vi "System@ErrorBox__Parameter.vi"(1 "ParamterIn":string) -> (0 "ParamterOut":string)   [LabVIEW 2020]
panel:
  in  "LogMessage":string(combo)
  in  "UserMessage":string(combo)
  in  "Logic":string(combo)
  in  "Confirm":bool
  # "System@ErrorBox $Logic,$UserMessage(,$LogMessage)"
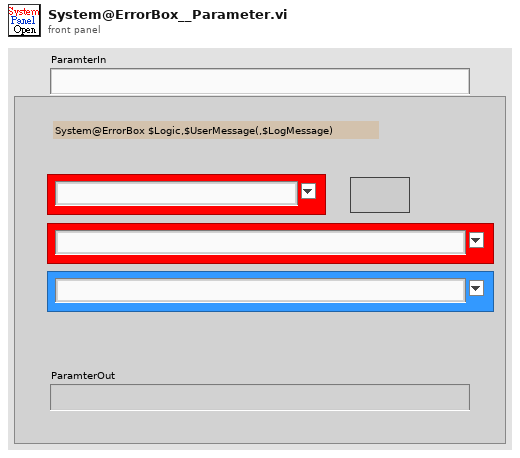
[diagram p1: front panel]
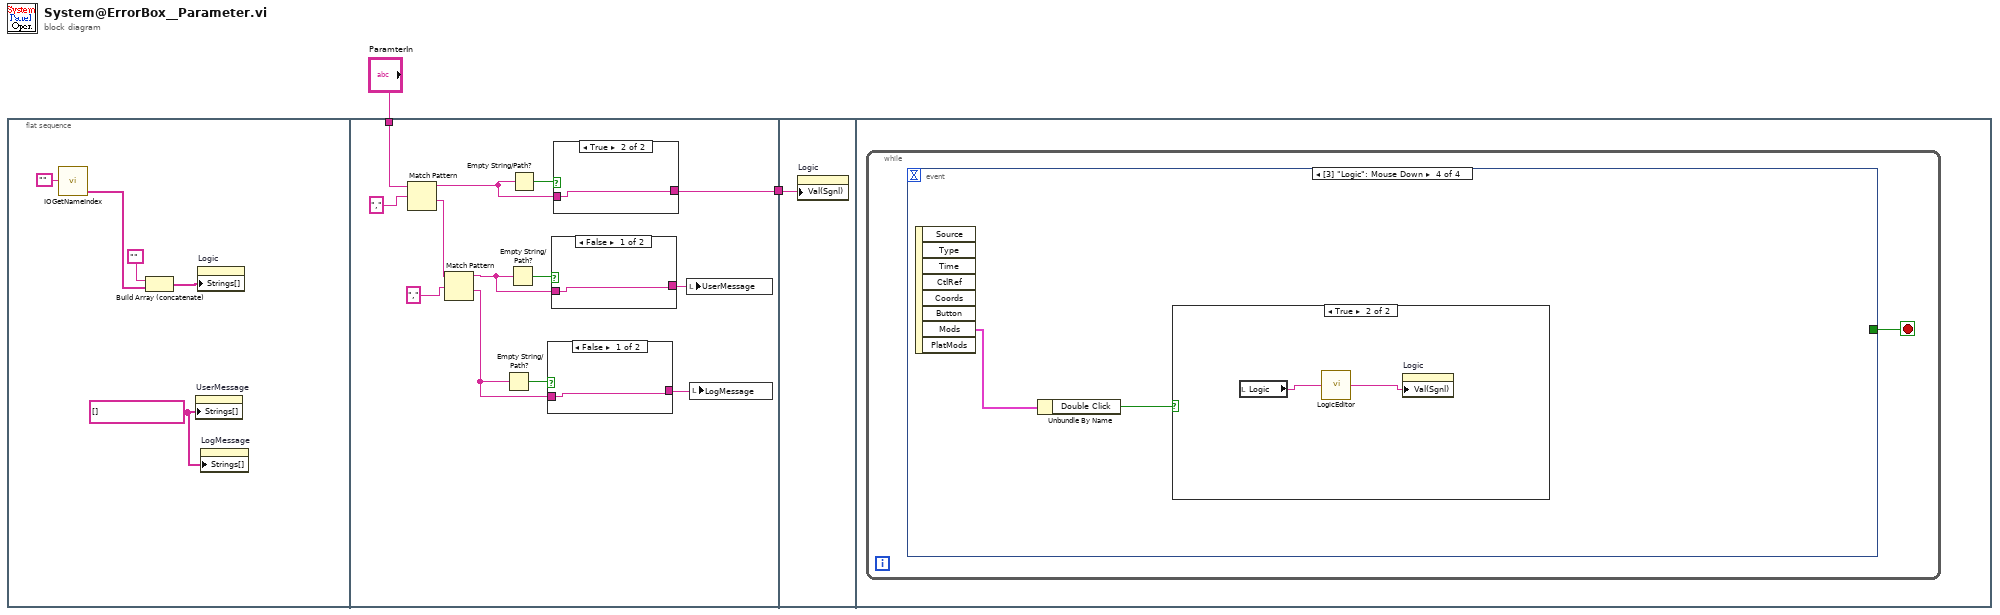
[diagram p0: block diagram]
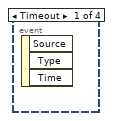
[diagram p5: hidden frame]
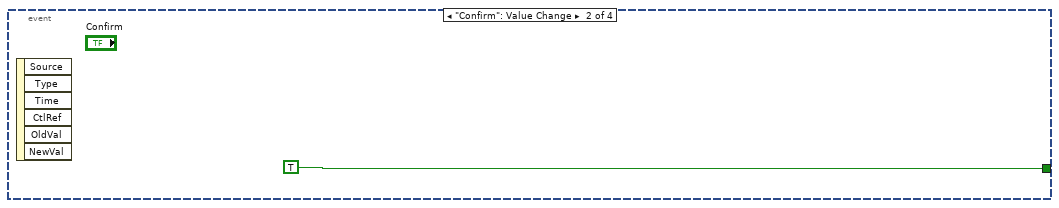
[diagram p6: hidden frame]
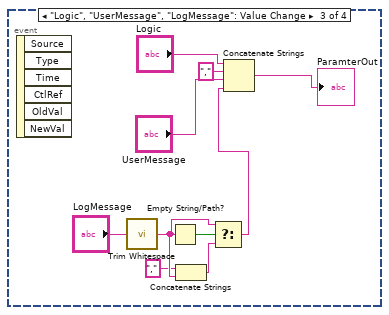
[diagram p7: hidden frame]
diagram:
  n1 = flat-sequence {
    tunnel: "ParamterIn" -> [w19]
    tunnel: [w15] -> w1
    tunnel: w1 -> [w27]
    frame #0 {
      w3 = string[] [] ("Strings []")
      n2 = call "IOGetNameIndex.vi"("PortName"="") -> ("PortNameList Out"=w6:string[])  [unwired: 3 in, 1 out]
      n3 = Build Array (concatenate)("", w6) -> (w4:string[])
      n4 = property on="UserMessage" class="CmbBox"("Strings[]"=w3) -> ()  [unwired: 2 in, 2 out]
      n5 = property on="Logic" class="CmbBox"("Strings[]"=w4) -> ()  [unwired: 2 in, 2 out]
      n6 = property on="LogMessage" class="CmbBox"("Strings[]"=w3) -> ()  [unwired: 2 in, 2 out]
    }
    frame #1 {
      n7 = Match Pattern(string=w19, regular expression=",") -> (before substring=w17:string, after substring=w12:string)  [unwired: 1 in, 2 out]
      n8 = Match Pattern(string=w12, regular expression=",") -> (before substring=w11:string, after substring=w9:string)  [unwired: 1 in, 2 out]
      n9 = Empty String/Path?(string/path=w9) -> (empty?=w10:bool)
      n10 = Empty String/Path?(string/path=w11) -> (empty?=w16:bool)
      n11 = Empty String/Path?(string/path=w17) -> (empty?=w20:bool)
      n12 = case shown="False" w10 {
        tunnel: w9 -> [w21 w22]
        tunnel: [w21 w22] -> w8
        frame False {
        }
        frame True {
        }
      }
      n13 = case shown="False" w16 {
        tunnel: w11 -> [w23 w24]
        tunnel: [w23 w24] -> w14
        frame False {
        }
        frame True {
        }
      }
      n14 = case shown="True" w20 {
        tunnel: w17 -> [w25 w26]
        tunnel: [w25 w26] -> w15
        frame False {
        }
        frame True {
        }
      }
      n15 = local write "UserMessage"(w14) -> ()
      n16 = local write "LogMessage"(w8) -> ()
    }
    frame #2 {
      n17 = property on="Logic" class="CmbBox"("Val(Sgnl)"=w27) -> ()  [unwired: 2 in, 2 out]
    }
    frame #3 {
      n18 = while {
        stop <- w28 stop-if-true
        n19 = event shown="[3] \"Logic\": Mouse Down" {
          selector: _ -> [_ _ _ _]
          dyn-events: _ -> [_ _ _ _]
          timeout: _ -> [_ _ _ _]
          tunnel: [_ TRUE _ _] -> w28
          event Timeout {
            n20 = event-data() -> ()  [unwired: 1 in, 3 out]
          }
          event "Confirm": Value Change {
            n21 = event-data() -> ()  [unwired: 1 in, 6 out]
          }
          event "Logic", "UserMessage", "LogMessage": Value Change {
            n22 = event-data() -> ()  [unwired: 1 in, 6 out]
            n23 = call <vilib>:"Trim Whitespace.vi"("string"="LogMessage") -> ("trimmed string"=w33:string)  [unwired: 1 in]
            n24 = Empty String/Path?(string/path=w33) -> (empty?=w34:bool)
            n25 = Concatenate Strings("," ("string"), w33) -> (w31:string)
            n26 = Select(t=w33, s=w34, f=w31) -> (s? t:f=w30:string)
            n27 = Concatenate Strings("Logic", "," ("string"), "UserMessage", w30) -> (→"ParamterOut":string)
          }
          event "Logic": Mouse Down {
            n28 = event-data() -> ("Mods"=w41:cluster{"Double Click":bool, "Menu Key":bool})  [unwired: 1 in, 7 out]
            n29 = Unbundle By Name(w41) -> ("Double Click"=w40:bool)
            n30 = case shown="True" w40 {
              frame False {
              }
              frame True {
                n31 = local read "Logic"() -> (w43:string)
                n32 = call "LogicEditor.vi"("Logic Express"=w43) -> ("LogicExpressOut"=w42:string)
                n33 = property on="Logic" class="CmbBox"("Val(Sgnl)"=w42) -> ()  [unwired: 2 in, 2 out]
              }
            }
          }
        }
      }
    }
  }
